vi "LVClass_Camera Reset to Factory CameraSet.vi"(0 "Camera in":refnum<class "Camera.lvclass">, 5 "load_and_apply_connection_params":bool, 7 "load_and_apply_params":bool, 11 "error in (no error)":errorcluster) -> (4 "Camera out":refnum<class "Camera.lvclass">, 15 "error out":errorcluster)   [LabVIEW 2020, in "Camera.lvclass"]
doc: "Reset camera parameters to factory values.\n\n<B>CameraIn</B> : Camera object.\n<B>CameraOut</B> : Camera object.\n<B>reset_connection_params</B> : try to load and apply factory connection parameters if true\n<B>reset_params</B> : try to load and apply factory parameters if true."
uses:
  Camera.lvclass
  Camera.lvclass/Camera.ctl
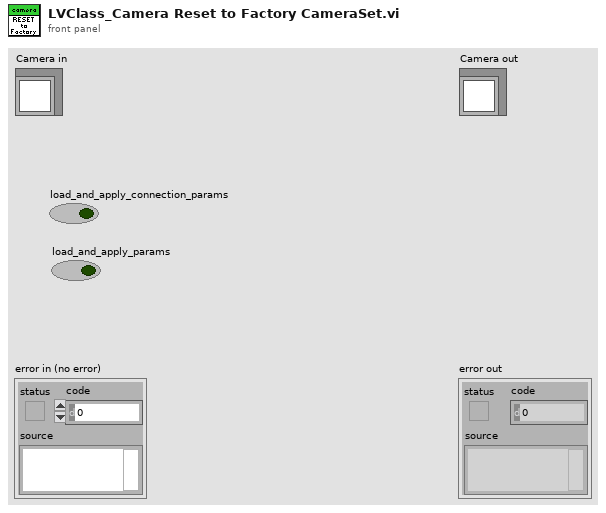
[diagram p1: front panel]
types:
  T1 = typedef "ClassID.ctl" = i64
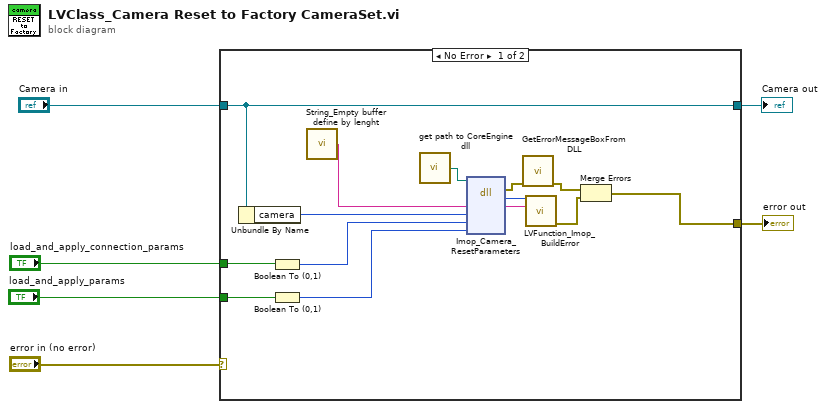
[diagram p0: block diagram]
diagram:
  n1 = case shown="No Error" "error in (no error)" {
    selector: "error in (no error)" -> [_ w22]
    tunnel: [w19 w22] -> w5
    tunnel: [w18 w21] -> w3
    tunnel: "Camera in" -> [w18 w21]
    tunnel: "load_and_apply_connection_params" -> [w10 _]
    tunnel: "load_and_apply_params" -> [w9 _]
    frame No Error {
      n2 = Unbundle By Name(w18) -> ("camera"=w17:T1)
      n3 = Boolean To (0,1)(Boolean=w10) -> (0, 1=w7:i16)
      n4 = Boolean To (0,1)(Boolean=w9) -> (0, 1=w8:i16)
      n5 = call "String_Empty buffer define by lenght.vi"() -> ("Empty buffer"=w20:string)  [unwired: 1 in]
      n6 = call "get path to CoreEngine dll.vi"() -> ("path to wavekit library"=w14:path)  [unwired: 14 in, 1 out]
      n7 = dll-call lib="D:/soft/HASO_v3/SVN_trunk/ImOpCoreEngine4_LV2011/DLLs/c_interface_vc100.dll" fn="Imop_Camera_ResetParameters"(path in=w14, "message"=w20, "camera"=w17, "load_and_apply_connection_params"=w7, "load_and_apply_params"=w8) -> (error out=w13:errorcluster, "return type"=w15:i32, "message"=w16:string)  [unwired: 5 in, 1 out]
      n8 = call "GetErrorMessageBoxFromDLL.vi"("error IN"=w13) -> ("error OUT"=w12:errorcluster)  [unwired: 10 in]
      n9 = call "LVFunction_Imop_BuildError.vi"("code"=w15, "String to Prepend to source (\"\")"=w16) -> ("error out"=w11:errorcluster)  [unwired: 13 in]
      n10 = Merge Errors(w12, w11) -> (w19:errorcluster)
    }
    frame Error {
    }
  }
  "error out" <- w5
  "Camera out" <- w3
